vi "Cleanup Host Stream.vi"(8 "error in (no error)":errorcluster, 11 "Refs":T1) -> (0 "error out":errorcluster)   [LabVIEW 2019, in "CAN Stream Support Workspace Shared.lvlib"]
uses:
  CAN Stream Support Workspace Shared.lvlib
  Types/Host Stream Refs.ctl
  <vilib>/xnet/xnet.llb/XNET CAN Comm.ctl
  <vilib>/xnet/xnet.llb/XNET CAN Comm State.ctl
  <vilib>/xnet/xnet.llb/XNET CAN Last Err.ctl
  <vilib>/xnet/xnet.llb/XNET Frame CAN.ctl
  <vilib>/xnet/xnet.llb/XNET Frame Type CAN.ctl
  <vilib>/ErrorRing/Error Ring.xnode
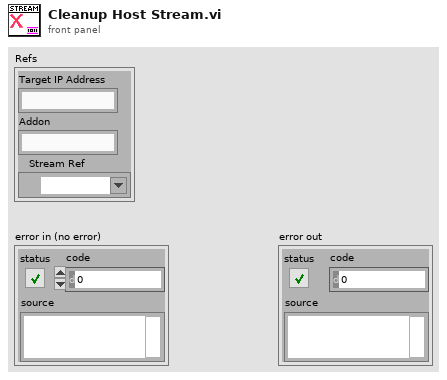
[diagram p1: front panel]
types:
  T1 = typedef "CAN Stream Support Workspace Shared.lvlib/Host Stream Refs.ctl" = cluster{"Target IP Address":string, "Addon":string, "Stream Ref":refnum<k21>}
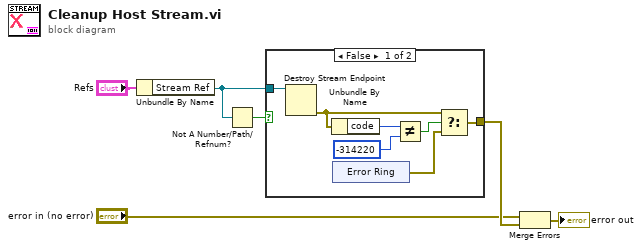
[diagram p0: block diagram]
diagram:
  n1 = Unbundle By Name("Refs") -> ("Stream Ref"=w1:refnum<k21>)
  n2 = Not A Number/Path/Refnum?(number/path/refnum=w1) -> (NaN/Path/Refnum?=w2:bool)
  n3 = case shown="False" w2 {
    tunnel: w1 -> [w13 _]
    tunnel: [w7 _] -> w5
    frame False {
      n4 = Destroy Stream Endpoint(11:w13) -> (0:w11:errorcluster)  [unwired: 1 in]
      n5 = Unbundle By Name(w11) -> ("code"=w8:i32)
      n6 = xnode "Error Ring"() -> ("error out"=w12:errorcluster)
      n7 = Not Equal?(x=w8, y=-314220) -> (x != y?=w10:bool)
      n8 = Select(t=w11, s=w10, f=w12) -> (s? t:f=w7:errorcluster)
    }
    frame True {
    }
  }
  n9 = Merge Errors("error in (no error)", w5) -> (→"error out":errorcluster)
